vi "Get Desired Size.vi"(8 "error in (no error)":errorcluster, 11 "ArrayPanel in":refnum<class "ArrayPanel.lvclass">) -> (0 "error out":errorcluster, 2 "Desired Size":T1, 3 "ArrayPanel out":refnum<class "ArrayPanel.lvclass">)   [LabVIEW 2020, in "OOPanel.lvlib" / "ArrayPanel.lvclass"]
uses:
  ArrayPanel.lvclass
  Desired Size.ctl
  OOPanel.lvlib
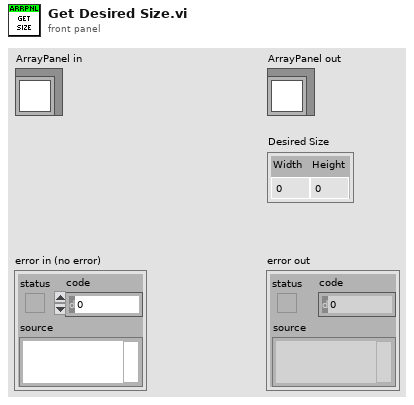
[diagram p1: front panel]
types:
  T1 = typedef "OOPanel.lvlib/Desired Size.ctl" = cluster{"Width":u32, "Height":u32}
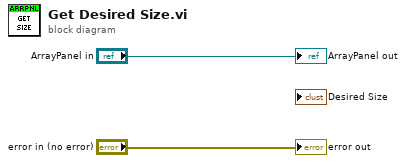
[diagram p0: block diagram]
diagram:
  "error out" <- "error in (no error)"
  "ArrayPanel out" <- "ArrayPanel in"
